vi "testOfariLogger.vi"   [LabVIEW 2020]
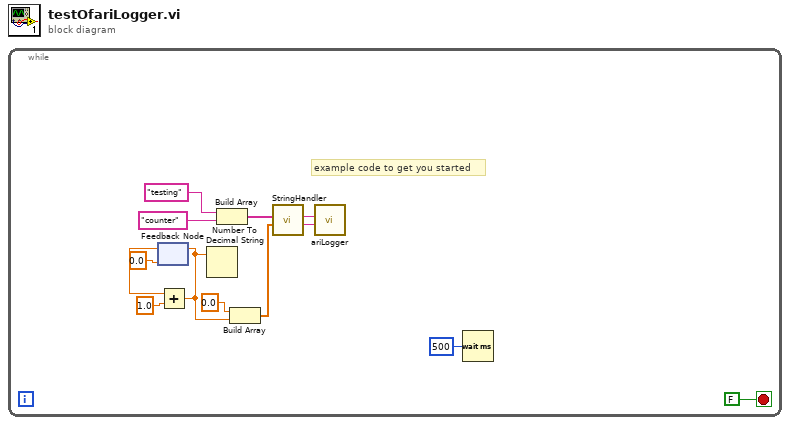
[diagram p0: block diagram]
diagram:
  n1 = while {
    stop <- FALSE stop-if-true
    # "example code to get you started"
    n2 = feedback #1(0.0 ("x")) -> (w11:dbl)
    n3 = Add(x=w11, y=1.0) -> (x+y=w4:dbl)
    n4 = feedback-in #1(w4) -> ()
    n5 = Number To Decimal String(number=w4) -> ()  [unwired: 1 in, 1 out]
    n6 = Build Array("testing", "counter" ("element")) -> (w8:string[])
    n7 = Build Array(0.0 ("element"), w4) -> (w3:dbl[])
    n8 = call "StringHandler.vi"("Data"=w3, "Names"=w8) -> ("Input"=w1:string, "Header"=w2:string)  [unwired: 8 in]
    n9 = call "ariLogger.vi"("Input"=w1, "Header"=w2) -> ()  [unwired: 10 in]
    n10 = Wait (ms)(milliseconds to wait=u32 500) -> ()  [unwired: 1 out]
  }
